vi "arduino_mvrel.vi"(8 "error in (no error)":errorcluster, 10 "steps":i32=100, 11 "VISA input":refnum<visa-resource-name>="COM8") -> (0 "error out":errorcluster, 2 "response":string="\n", 3 "VISA out":refnum<visa-resource-name>="COM8")   [LabVIEW 2017]
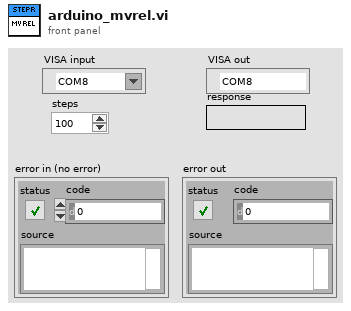
[diagram p1: front panel]
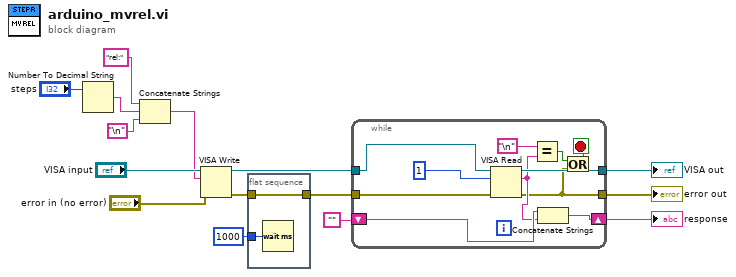
[diagram p0: block diagram]
diagram:
  n1 = Number To Decimal String(number="steps") -> (decimal integer string=w13:string)  [unwired: 1 in]
  n2 = Concatenate Strings("rel:" ("string"), w13, "\n") -> (w12:string)
  n3 = VISA Write(VISA resource name="VISA input", write buffer=w12, error in (no error)="error in (no error)") -> (VISA resource name out=w9:refnum<visa-resource-name>, error out=w3:errorcluster)  [unwired: 1 out]
  n4 = flat-sequence {
    tunnel: w3 -> [w17]
    tunnel: [w17] -> w2
    tunnel: 1000 -> [w16]
    frame #0 {
      n5 = Wait (ms)(milliseconds to wait=w16) -> ()  [unwired: 1 out]
    }
  }
  n6 = while {
    tunnel: w9 -> [w19]
    tunnel: w2 -> [w20]
    shift-right: [w28] -> w5
    shift-left: "" -> [w25]
    tunnel: [w22] -> w6
    tunnel: [w26] -> w7
    stop <- w21 stop-if-true
    n7 = VISA Read(VISA resource name=w19, byte count=u32 1, error in (no error)=w20) -> (VISA resource name out=w26:refnum<visa-resource-name>, read buffer=w24:string, error out=w22:errorcluster)  [unwired: 1 out]
    n8 = Equal?(x="\n", y=w24) -> (x = y?=w23:bool)
    n9 = Concatenate Strings(w25, w24) -> (w28:string)
    n10 = Or(x=w23, y=w22) -> (x .or. y?=w21:bool)
  }
  "VISA out" <- w7
  "error out" <- w6
  "response" <- w5
